vi "基础22.vi"() -> ()   [LabVIEW 2014]
uses:
  <vilib>/Utility/file.llb/Write To Spreadsheet File (string).vi
panel:
  in  "停止":bool
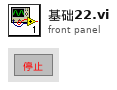
[diagram p1: front panel]
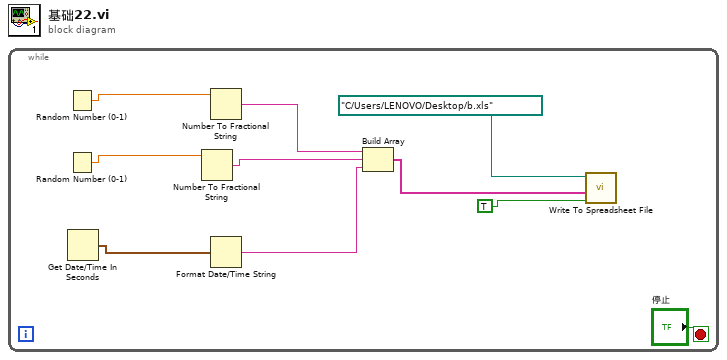
[diagram p0: block diagram]
diagram:
  n1 = while {
    stop <- "停止" stop-if-true
    n2 = Random Number (0-1)() -> (number: 0 to 1=w4:dbl)
    n3 = Random Number (0-1)() -> (number: 0 to 1=w3:dbl)
    n4 = Get Date/Time In Seconds() -> (seconds since 1Jan1904=w10:timestamp)
    n5 = Number To Fractional String(number=w3) -> (F-format string=w1:string)  [unwired: 3 in]
    n6 = Number To Fractional String(number=w4) -> (F-format string=w2:string)  [unwired: 3 in]
    n7 = Format Date/Time String(seconds (now)=w10) -> (date/time string=w9:string)  [unwired: 2 in]
    n8 = Build Array(w2, w1, w9) -> (w7:string[])
    n9 = call-poly <vilib>:"Write To Spreadsheet File.vi"("append to file? (new file:F)"=TRUE, "1D data"=w7, "file path (dialog if empty)"=path "C:/Users/LENOVO/Desktop/b.xls") -> ()  [unwired: 5 in, 1 out]
  }
